vi "overlay_+[].vi"(7 "CCD编号":T2 items=["空", "CCD0", "CCD1", "CCD2", "CCD3", "CCD4", "CCD5", "CCD6", "CCD7"], 10 "ROI Descriptor":T1 {"Contours"."Type" items=["No Selection", "Point", "Line", "Rectangle", "Oval", "Polygon", "Freehand Region", "Annulus", "Unused2", "Unused3", "Broken Line", "Freehand Line", "Rotated Rectangle"]}, 11 "Image":T3) -> (3 "Imageout":T3)   [LabVIEW 2014]
uses:
  <vilib>/vision/Image Controls.llb/IMAQ Image.ctl
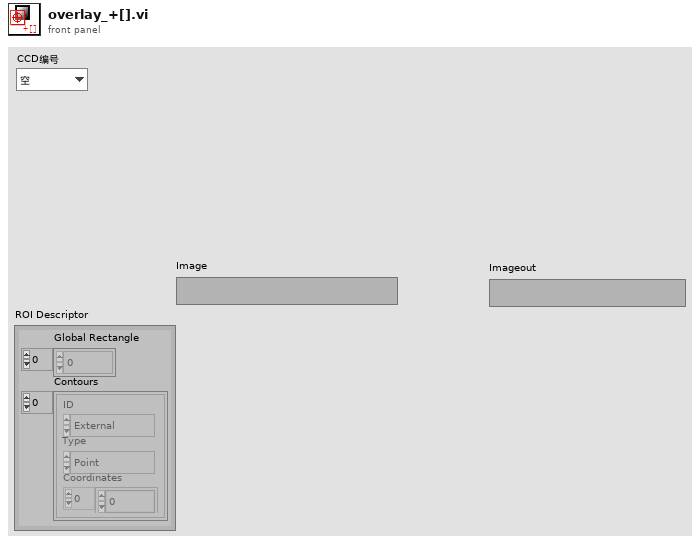
[diagram p1: front panel]
types:
  T1 = typedef "ROI Descriptor" = cluster{"Global Rectangle":i32[], "Contours":cluster{"ID":enum32{"External", "Internal"}, "Type":u32, "Coordinates":i32[]}[]}
  T2 = typedef "ccd编号.ctl" = u16
  T3 = typedef "IMAQ Image.ctl" = refnum<image>
  T4 = typedef "工序1机种参数.ctl" = cluster{"屏大小":cluster{"X":dbl, "Y":dbl, "Z":dbl}, "壳大小":cluster{"X":dbl, "Y":dbl, "Z":dbl}, "CCD0通用亮度":T5, "CCD1通用亮度":T5, "V_XY":dbl, "ACC_XY":dbl, "V_Z":dbl, "ACC_Z":dbl, "V_C":dbl, "ACC_C":dbl, "V_B":dbl, "ACC_B":dbl, "识别异常处理方式":cluster{"模式":enum16{"立即报警", "连续N次异常报警"}, "抛料N次后报警":dbl}}
  T5 = typedef "Light.ctl" = cluster{"L1":dbl, "L2":dbl, "L3":dbl, "L4":dbl}
  T6 = enum16{"open", "save", "read", "write", "savedefault", "readdefault"}
  T7 = typedef "CCD NO..ctl" = cluster{"CCD编号":T2, "ccd config":T8}
  T8 = typedef "ccd config.ctl" = cluster{"Session In":T9, "Image Size":cluster{"x":i32, "y":i32}, "Type of Symmetry":u32, "Angle (degrees)":sgl, "Image Center":cluster{"x":i32, "y":i32}, "光源串口":T10}
  T9 = typedef "IMAQdx.ctl" = refnum<k21>
  T10 = typedef "光源串口.ctl" = T11[]
  T11 = typedef "串口.ctl" = cluster{"名称":u16, "串口":T12}
  T12 = typedef "串口base.ctl" = cluster{"COM":refnum<visa-resource-name>, "数据位":u16, "波特率":u32, "停止位":u16, "控制流":u16, "奇偶校验":enum16{"None", "Odd", "Even", "Mark", "Space"}}
  T13 = typedef "IMAQ Rectangle" = cluster{"Left":i32, "Top":i32, "Right":i32, "Bottom":i32, "Rotation":dbl}
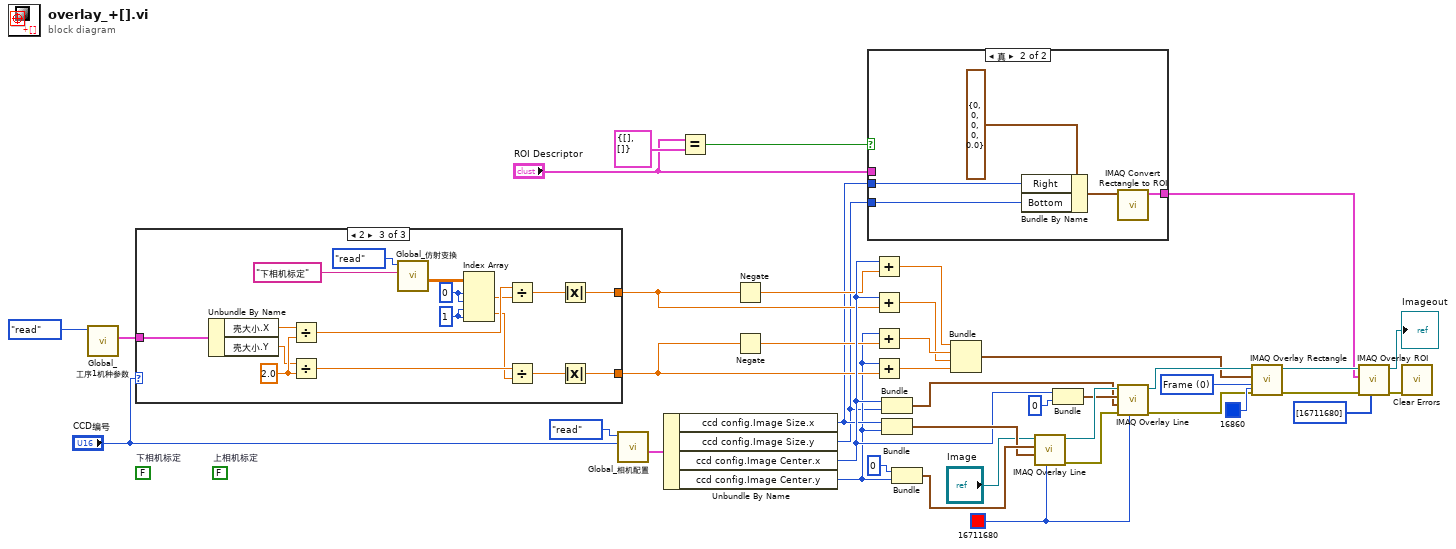
[diagram p0: block diagram]
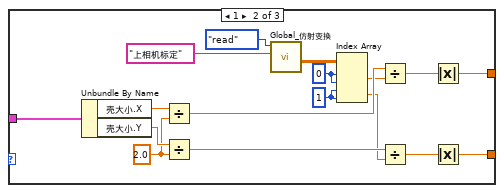
[diagram p4: hidden frame]
diagram:
  (unwired) FALSE  # 下相机标定
  (unwired) FALSE  # 上相机标定
  w26 = u32 0 items=["Frame", "Fill", "Highlight"] ("Drawing Mode (Frame)")
  w31 = u32 16711680 ("Color")
  n1 = call "Global_工序1机种参数.vi"("操作"=enum16{"open", "read", "save"}."read") -> ("工序1机种参数"=w28:T4)  [unwired: 10 in]
  n2 = case shown="2" "CCD编号" {
    tunnel: w28 -> [_ w58 w75]
    tunnel: [_ w42 w60] -> w21
    tunnel: [_ w43 w59] -> w23
    frame 0, Default {
    }
    frame 1 {
      w45 = 1 ("索引 (行)")
      w51 = 0 ("索引 (行)")
      w55 = 2.0 ("y")
      n3 = Unbundle By Name(w58) -> ("壳大小.X"=w57:dbl, "壳大小.Y"=w56:dbl)
      n4 = Divide(x=w57, y=w55) -> (x/y=w49:dbl)
      n5 = Divide(x=w56, y=w55) -> (x/y=w46:dbl)
      n6 = call "Global_仿射变换.vi"("name"="上相机标定", "操作"=T6."read") -> ("变换关系out"=w52:dbl[][])  [unwired: 8 in, 1 out]
      n7 = Index Array(array=w52, index (row) #1=w51, index (col) #1=w51, index (row) #2=w45, index (col) #2=w45) -> (element #1=w48:dbl, element #2=w44:dbl)
      n8 = Divide(x=w49, y=w48) -> (x/y=w50:dbl)
      n9 = Divide(x=w46, y=w44) -> (x/y=w47:dbl)
      n10 = Absolute Value(x=w50) -> (abs(x)=w42:dbl)
      n11 = Absolute Value(x=w47) -> (abs(x)=w43:dbl)
    }
    frame 2 {
      w64 = 1 ("索引 (行)")
      w69 = 0 ("索引 (行)")
      w74 = 2.0 ("y")
      n12 = Unbundle By Name(w75) -> ("壳大小.X"=w73:dbl, "壳大小.Y"=w72:dbl)
      n13 = Divide(x=w73, y=w74) -> (x/y=w66:dbl)
      n14 = Divide(x=w72, y=w74) -> (x/y=w62:dbl)
      n15 = call "Global_仿射变换.vi"("name"="下相机标定", "操作"=T6."read") -> ("变换关系out"=w68:dbl[][])  [unwired: 8 in, 1 out]
      n16 = Index Array(array=w68, index (row) #1=w69, index (col) #1=w69, index (row) #2=w64, index (col) #2=w64) -> (element #1=w65:dbl, element #2=w61:dbl)
      n17 = Divide(x=w66, y=w65) -> (x/y=w67:dbl)
      n18 = Divide(x=w62, y=w61) -> (x/y=w63:dbl)
      n19 = Absolute Value(x=w67) -> (abs(x)=w60:dbl)
      n20 = Absolute Value(x=w63) -> (abs(x)=w59:dbl)
    }
  }
  n21 = call "Global_相机配置.vi"("CCD编号"="CCD编号", "枚举"=enum16{"read", "write", "open", "save"}."read") -> ("CCDCFGOUT"=w40:T7)  [unwired: 8 in, 1 out]
  n22 = Unbundle By Name(w40) -> ("ccd config.Image Size.x"=w3:i32, "ccd config.Image Size.y"=w1:i32, "ccd config.Image Center.x"=w24:i32, "ccd config.Image Center.y"=w2:i32)
  n23 = Equal?(x="ROI Descriptor", y=T1 {"Global Rectangle"=[], "Contours"=[]}) -> (x = y?=w6:bool)
  n24 = Negate(x=w21) -> (-x=w20:dbl)
  n25 = Negate(x=w23) -> (-x=w22:dbl)
  n26 = case shown="真" w6 {
    tunnel: [w76 w79] -> w5
    tunnel: "ROI Descriptor" -> [w76 _]
    tunnel: w3 -> [_ w78]
    tunnel: w1 -> [_ w77]
    frame False {
    }
    frame True {
      n27 = Bundle By Name(cluster=T13 {"Left"=0, "Top"=0, "Right"=0, "Bottom"=0, "Rotation"=0.0} ("Rectangle"), "Right"=w78, "Bottom"=w77) -> (w80:T13)
      n28 = call "IMAQ Convert Rectangle to ROI"("Rectangle"=w80) -> ("ROI Descriptor"=w79:T1)  [unwired: 8 in, 1 out]
    }
  }
  n29 = Add(x=w24, y=w20) -> (x+y=w19:dbl)
  n30 = Add(x=w24, y=w21) -> (x+y=w17:dbl)
  n31 = Add(x=w2, y=w22) -> (x+y=w18:dbl)
  n32 = Add(x=w2, y=w23) -> (x+y=w16:dbl)
  n33 = Bundle("x"=w24, "y"=w1) -> (w32:cluster{"x":i32, "y":i32})  [unwired: 1 in]
  n34 = Bundle("x"=w3, "y"=w2) -> (w36:cluster{"x":i32, "y":i32})  [unwired: 1 in]
  n35 = Bundle(0, "y"=w2) -> (w37:cluster{i32, "y":i32})  [unwired: 1 in]
  n36 = Bundle(w19, w18, w17, w16) -> (w15:cluster{dbl, dbl, dbl, dbl})  [unwired: 1 in]
  n37 = call "IMAQ Overlay Line"("Color"=w31, "End Point"=w36, "Start Point"=w37, "Image"="Image") -> ("error out"=w14:errorcluster, "Image Out"=w34:T3)  [unwired: 6 in]
  n38 = Bundle("x"=w24, 0) -> (w33:cluster{"x":i32, i32})  [unwired: 1 in]
  n39 = call "IMAQ Overlay Line"("Color"=w31, "error in (no error)"=w14, "End Point"=w32, "Start Point"=w33, "Image"=w34) -> ("error out"=w13:errorcluster, "Image Out"=w27:T3)  [unwired: 5 in]
  n40 = call "IMAQ Overlay Rectangle"("Color"=u32 16860, "error in (no error)"=w13, "Drawing Mode (Frame)"=w26, "Rectangle"=w15, "Image"=w27) -> ("error out"=w12:errorcluster, "Image Out"=w10:T3)  [unwired: 5 in]
  n41 = call "IMAQ Overlay ROI"("Colors (Green)"=u32[] [16711680], "error in (no error)"=w12, "ROI Descriptor"=w5, "Image"=w10) -> ("error out"=w11:errorcluster, "Image Out"=→"Imageout":T3)  [unwired: 6 in]
  n42 = call <vilib>:"Clear Errors.vi"("error in (no error)"=w11) -> ()  [unwired: 5 in, 2 out]
